vi "Room to Hallway.vi"(8 "error in (no error)":errorcluster, 10 "LRU Cache in":refnum<class "LRU Cache.lvclass">, 11 "State in":refnum<class "State.lvclass">) -> (0 "error out":errorcluster, 2 "LRU Cache out":refnum<class "LRU Cache.lvclass">, 3 "State out":refnum<class "State.lvclass">)   [LabVIEW 2019, in "23.lvlib" / "State.lvclass"]
uses:
  State.lvclass
  C:/Users/craig.walker/Documents/GitHub/lv2019-LRU-Cache/LRU Node/LRU Node.lvclass
  lv2019-LRU-Cache/LRU Cache/LRU Cache.lvclass
  lv2019-LRU-Cache/LRU Node/LRU Node.lvclass/LRU Node.ctl
  State Value/State Value.lvclass/State Value.ctl
  State Key/State Key.lvclass/State Key.ctl
  lv2019-LRU-Cache/LRU Node/Write Value.vi
  lv2019-LRU-Cache/LRU Node/Read Value.vi
  Between.vi
  lv2019-LRU-Cache/LRU Node/Read Key.vi
  lv2019-LRU-Cache/LRU Node/Write Key.vi
  State Value/State Value.lvclass
  State Key/State Key.lvclass
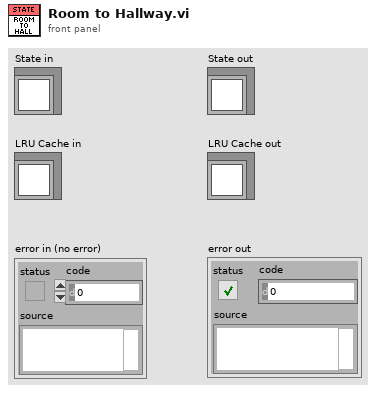
[diagram p1: front panel]
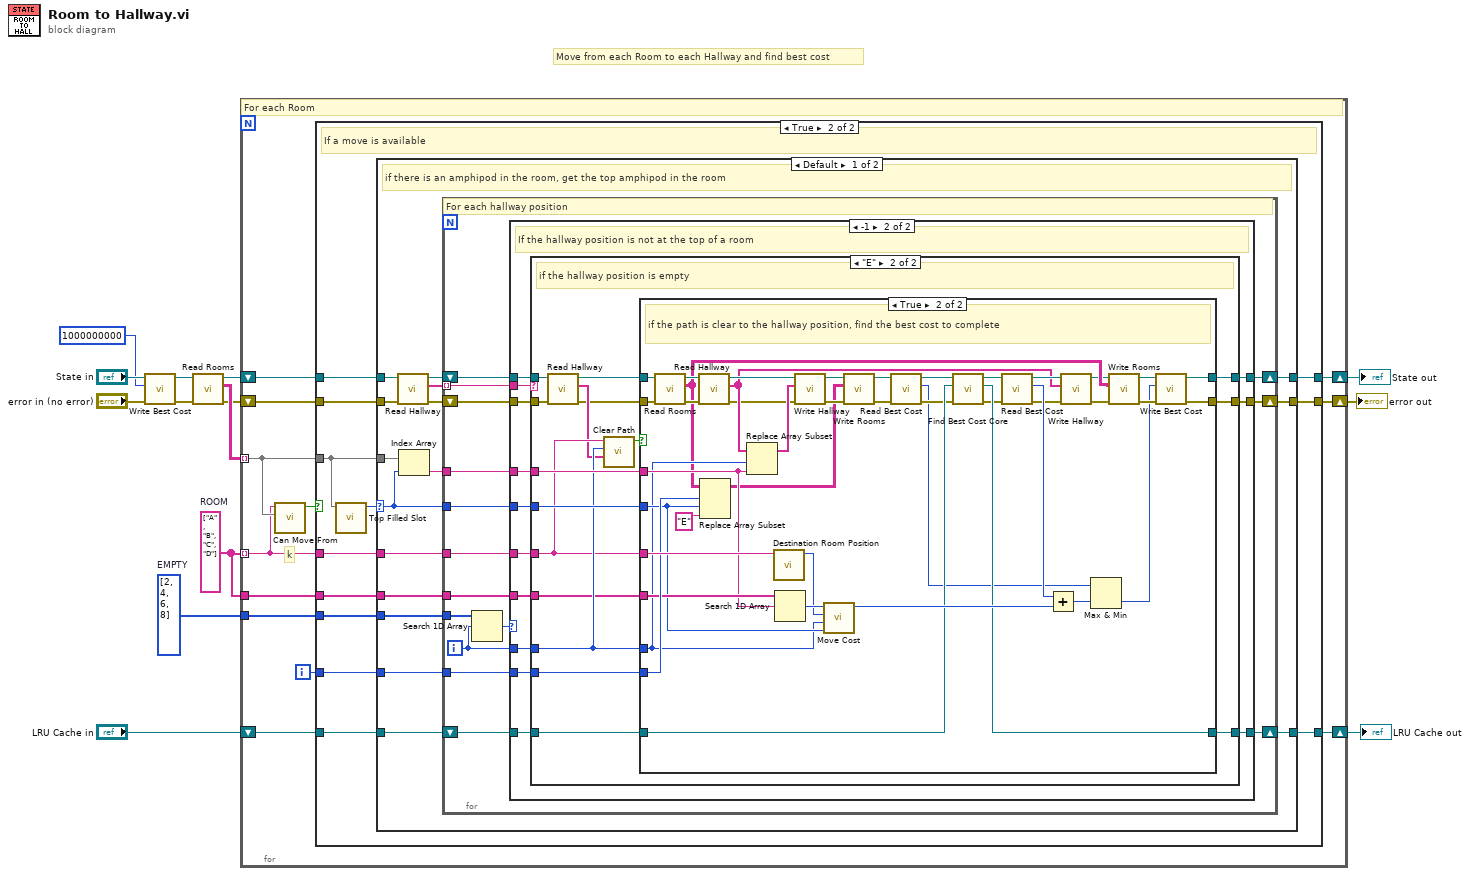
[diagram p0: block diagram]
diagram:
  w13 = string[] ["A", "B", "C", "D"]  # ROOM
  w14 = u64[] [2, 4, 6, 8]  # EMPTY
  # "Move from each Room to each Hallway and find best cost"
  n1 = call "Write Best Cost.vi"("error in (no error)"="error in (no error)", "Best Cost"=u64 1000000000, "State in"="State in") -> ("error out"=w3:errorcluster, "State out"=w9:refnum<class "State.lvclass">)  [unwired: 7 in]
  n2 = call "Read Rooms.vi"("error in (no error)"=w3, "State in"=w9) -> ("error out"=w2:errorcluster, "Rooms"=w5:string[][], "State out"=w6:refnum<class "State.lvclass">)  [unwired: 7 in]
  n3 = for {
    tunnel: w5 -> [w25] mode=indexing
    tunnel: w13 -> [w24] mode=indexing
    tunnel: w14 -> [w22]
    tunnel: w13 -> [w21]
    shift-right: [w19] -> w11
    shift-left: "LRU Cache in" -> [w20]
    shift-right: [w17] -> w7
    shift-left: w6 -> [w18]
    shift-right: [w15] -> w1
    shift-left: w2 -> [w16]
    i -> [w23]
    # "k"
    # "For each Room"
    n4 = call "Can Move From.vi"("Room"=w25, "Amphipod"=w24) -> ("Can Move From?"=w26:bool)  [unwired: 9 in]
    n5 = case shown="True" w26 {
      tunnel: w25 -> [_ w40]
      tunnel: w22 -> [_ w39]
      tunnel: w24 -> [_ w38]
      tunnel: w23 -> [_ w37]
      tunnel: w21 -> [_ w36]
      tunnel: w20 -> [w29 w35]
      tunnel: [w29 w34] -> w19
      tunnel: w18 -> [w28 w33]
      tunnel: [w28 w32] -> w17
      tunnel: w16 -> [w27 w31]
      tunnel: [w27 w30] -> w15
      frame False {
        # "If a move is not available try the next room"
      }
      frame True {
        # "If a move is available"
        n6 = call "Top Filled Slot.vi"("Room"=w40) -> ("Top Filled Slot"=w41:i32)  [unwired: 10 in]
        n7 = case shown="Default" w41 {
          selector: w41 -> [w55 _]
          tunnel: w40 -> [w53 _]
          tunnel: w39 -> [w57 _]
          tunnel: w38 -> [w56 _]
          tunnel: w37 -> [w52 _]
          tunnel: w36 -> [w51 _]
          tunnel: w35 -> [w50 w155]
          tunnel: [w49 w155] -> w34
          tunnel: w33 -> [w48 w154]
          tunnel: [w44 w154] -> w32
          tunnel: w31 -> [w43 w153]
          tunnel: [w42 w153] -> w30
          frame Default {
            # "if there is an amphipod in the room, get the top amphipod in the room"
            n8 = call "Read Hallway.vi"("error in (no error)"=w43, "State in"=w48) -> ("error out"=w45:errorcluster, "Hallway"=w47:string[], "State out"=w46:refnum<class "State.lvclass">)  [unwired: 7 in]
            n9 = Index Array(array=w53, index=w55) -> (element=w54:string)
            n10 = for {
              tunnel: w47 -> [w70] mode=indexing
              tunnel: w57 -> [w72]
              tunnel: w56 -> [w69]
              tunnel: w55 -> [w67]
              tunnel: w54 -> [w66]
              tunnel: w52 -> [w65]
              tunnel: w51 -> [w64]
              shift-right: [w62] -> w49
              shift-left: w50 -> [w63]
              shift-right: [w60] -> w44
              shift-left: w46 -> [w61]
              shift-right: [w59] -> w42
              shift-left: w45 -> [w58]
              i -> [w68]
              # "For each hallway position"
              n11 = Search 1D Array(1D array=w72, element=w68) -> (index of element=w71:i32)  [unwired: 1 in]
              n12 = case shown="-1" w71 {
                tunnel: w70 -> [_ w88]
                tunnel: w69 -> [_ w87]
                tunnel: w68 -> [_ w86]
                tunnel: w67 -> [_ w85]
                tunnel: w66 -> [_ w84]
                tunnel: w65 -> [_ w83]
                tunnel: w64 -> [_ w82]
                tunnel: w63 -> [w75 w81]
                tunnel: [w75 w80] -> w62
                tunnel: w61 -> [w74 w79]
                tunnel: [w74 w78] -> w60
                tunnel: [w73 w77] -> w59
                tunnel: w58 -> [w73 w76]
                frame Default {
                  # "if the hallway position is at the top of a room try the next one"
                }
                frame -1 {
                  # "If the hallway position is not at the top of a room"
                  n13 = case shown="\"E\"" w88 {
                    tunnel: w87 -> [_ w103]
                    tunnel: w86 -> [_ w104]
                    tunnel: w85 -> [_ w106]
                    tunnel: w84 -> [_ w105]
                    tunnel: w83 -> [_ w102]
                    tunnel: w82 -> [_ w101]
                    tunnel: w81 -> [w91 w100]
                    tunnel: [w91 w99] -> w80
                    tunnel: w79 -> [w90 w98]
                    tunnel: [w90 w95] -> w78
                    tunnel: [w89 w94] -> w77
                    tunnel: w76 -> [w89 w93]
                    frame Default {
                      # "if the hallway position is filled, try the next one"
                    }
                    frame "E" {
                      # "if the hallway position is empty"
                      n14 = call "Read Hallway.vi"("error in (no error)"=w93, "State in"=w98) -> ("error out"=w92:errorcluster, "Hallway"=w97:string[], "State out"=w96:refnum<class "State.lvclass">)  [unwired: 7 in]
                      n15 = call "Clear Path.vi"("Hallway"=w97, "Hallway Position"=w104, "Room"=w103) -> ("Clear Path?"=w107:bool)  [unwired: 8 in]
                      n16 = case shown="True" w107 {
                        tunnel: w106 -> [_ w145]
                        tunnel: w105 -> [_ w147]
                        tunnel: w104 -> [_ w143]
                        tunnel: w103 -> [_ w152]
                        tunnel: w102 -> [_ w151]
                        tunnel: w101 -> [_ w149]
                        tunnel: w100 -> [w110 w141]
                        tunnel: [w110 w140] -> w99
                        tunnel: w96 -> [w108 w139]
                        tunnel: [w108 w118] -> w95
                        tunnel: [w109 w117] -> w94
                        tunnel: w92 -> [w109 w111]
                        frame False {
                        }
                        frame True {
                          # "if the path is clear to the hallway position, find the best cost to complete"
                          n17 = call "Read Rooms.vi"("error in (no error)"=w111, "State in"=w139) -> ("error out"=w137:errorcluster, "Rooms"=w124:string[][], "State out"=w138:refnum<class "State.lvclass">)  [unwired: 7 in]
                          n18 = call "Read Hallway.vi"("error in (no error)"=w137, "State in"=w138) -> ("error out"=w126:errorcluster, "Hallway"=w127:string[], "State out"=w135:refnum<class "State.lvclass">)  [unwired: 7 in]
                          n19 = Replace Array Subset(array=w124, new element="E" ("y"), index (row)=w151, index (col)=w145) -> (w132:string[][])
                          n20 = Replace Array Subset(array=w127, new element=w147, index=w143) -> (w136:string[])
                          n21 = call "Destination Room Position.vi"("Amphipod Type"=w152) -> ("Destination Room Position"=w144:i32)  [unwired: 10 in]
                          n22 = Search 1D Array(1D array=w149, element=w147) -> (index of element=w146:i32)  [unwired: 1 in]
                          n23 = call "Write Hallway.vi"("error in (no error)"=w126, "Hallway"=w136, "State in"=w135) -> ("error out"=w134:errorcluster, "State out"=w133:refnum<class "State.lvclass">)  [unwired: 7 in]
                          n24 = call "Move Cost.vi"("Room Slot"=w145, "Destination Position"=w143, "Source Position"=w144, "Amphipod Type Index"=w146) -> ("Move Cost"=w142:u64)  [unwired: 7 in]
                          n25 = call "Write Rooms.vi"("error in (no error)"=w134, "Rooms"=w132, "State in"=w133) -> ("error out"=w114:errorcluster, "State out"=w116:refnum<class "State.lvclass">)  [unwired: 7 in]
                          n26 = call "Read Best Cost.vi"("error in (no error)"=w114, "State in"=w116) -> ("error out"=w113:errorcluster, "Best Cost"=w112:u64, "State out"=w115:refnum<class "State.lvclass">)  [unwired: 7 in]
                          n27 = call "Find Best Cost Core.vi"("error in (no error)"=w113, "LRU Cache in"=w141, "State in"=w115) -> ("error out"=w131:errorcluster, "LRU Cache out"=w140:refnum<class "LRU Cache.lvclass">, "State out"=w130:refnum<class "State.lvclass">)  [unwired: 6 in]
                          n28 = call "Read Best Cost.vi"("error in (no error)"=w131, "State in"=w130) -> ("error out"=w125:errorcluster, "Best Cost"=w129:u64, "State out"=w128:refnum<class "State.lvclass">)  [unwired: 7 in]
                          n29 = Add(x=w129, y=w142) -> (x+y=w148:u64)
                          n30 = call "Write Hallway.vi"("error in (no error)"=w125, "Hallway"=w127, "State in"=w128) -> ("error out"=w122:errorcluster, "State out"=w123:refnum<class "State.lvclass">)  [unwired: 7 in]
                          n31 = Max & Min(x=w112, y=w148) -> (min(x,y)=w119:u64)  [unwired: 1 out]
                          n32 = call "Write Rooms.vi"("error in (no error)"=w122, "Rooms"=w124, "State in"=w123) -> ("error out"=w120:errorcluster, "State out"=w121:refnum<class "State.lvclass">)  [unwired: 7 in]
                          n33 = call "Write Best Cost.vi"("error in (no error)"=w120, "Best Cost"=w119, "State in"=w121) -> ("error out"=w117:errorcluster, "State out"=w118:refnum<class "State.lvclass">)  [unwired: 7 in]
                        }
                      }
                    }
                  }
                }
              }
            }
          }
          frame -1 {
            # "if there is no amphipod in the room, try the next one"
          }
        }
      }
    }
  }
  "State out" <- w7
  "LRU Cache out" <- w11
  "error out" <- w1
